vi "EnableWFG.vi"(0 "object in":refnum<class "AFG3022B_OJ.lvclass">, 2 "Enable Output (T: Enable)":bool=TRUE, 3 "Channel (0: Channel 1)":u16(ring) items=["Channel 1", "Channel2"], 5 "error in (no error)":errorcluster) -> (14 "object out":refnum<class "AFG3022B_OJ.lvclass">, 19 "error out":errorcluster)   [LabVIEW 2023, in "AFG3022B_OJ.lvclass"]
uses:
  AFG3022B_OJ.lvclass
  AFG3022B_OJ.lvclass/AFG3022B_OJ.ctl
  PowerScan/Tektronix AFG 3000 Series/Tektronix AFG 3000 Series.lvlib
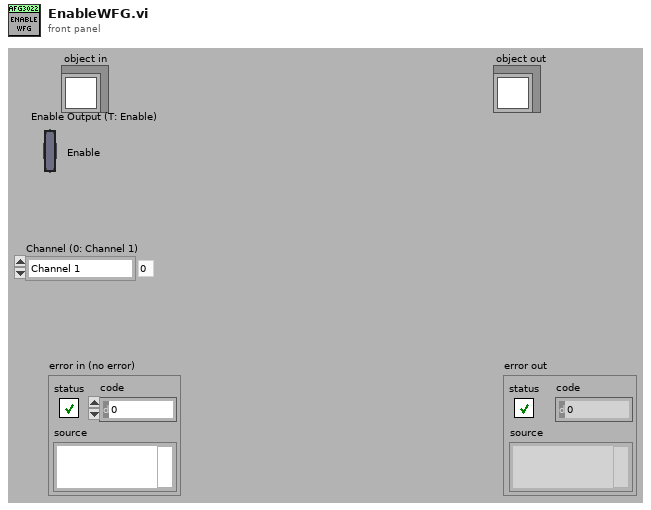
[diagram p1: front panel]
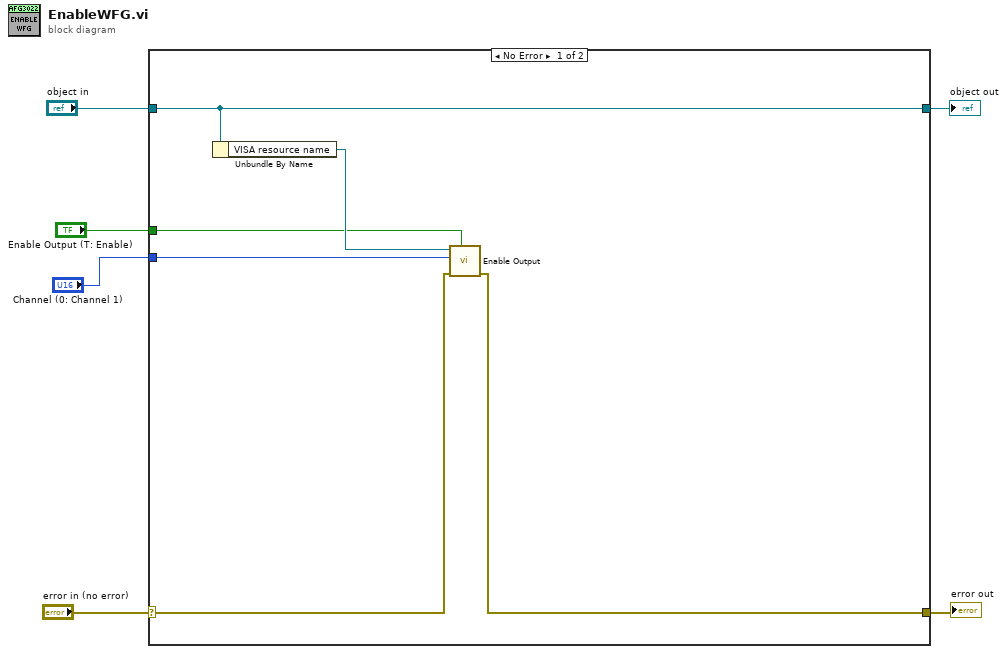
[diagram p0: block diagram]
diagram:
  n1 = case shown="No Error" "error in (no error)" {
    selector: "error in (no error)" -> [w8 w14]
    tunnel: [w7 w14] -> w5
    tunnel: [w12 w13] -> w3
    tunnel: "object in" -> [w12 w13]
    tunnel: "Enable Output (T: Enable)" -> [w10 _]
    tunnel: "Channel (0: Channel 1)" -> [w9 _]
    frame No Error {
      n2 = Unbundle By Name(w12) -> ("VISA resource name"=w11:refnum<visa-resource-name>)
      n3 = call "Enable Output.vi"("Enable Output (T: Enable)"=w10, "error in (no error)"=w8, "Channel (0: Channel 1)"=w9, "VISA resource name"=w11) -> ("error out"=w7:errorcluster)  [unwired: 6 in, 1 out]
    }
    frame Error {
    }
  }
  "error out" <- w5
  "object out" <- w3
